vi "Parallel Processing (Optimized Performance).vi"() -> ()   [LabVIEW 2023]
doc: "The Parallel Processing (Optimized Performance) example shows how to process multiple images in parallel when using a ring acquisition. Images acquired from a camera are stored in a ring buffer and references to each image are pushed to a queue. Each worker loop removes a reference from the queue and processes the image.\n\nIn this example, image processing is simulated by a time delay that can be adjusted while the VI is running. When processing is complete, <B>IMAQdx Release Image</B> must be called in order to free space in the ring buffer."
uses:
  <vilib>/vision/driver/IMAQdx.llb/IMAQdx Acquisition Mode.ctl
  <vilib>/vision/Image Controls.llb/IMAQ Image.ctl
  <vilib>/vision/driver/IMAQdx.llb/IMAQdx Buffer Number Mode.ctl
  <vilib>/vision/driver/NI_Vision_Acquisition_Software.lvlib
  <resource>/objmgr/imaqdx.rc
panel:
  out "Lost Buffer Count":u32
  in  "Processing Delay (s)":dbl(slide)=0.1 scale=0.0..1.0
  out "Images Processed":u32
  out "Current Buffer Number":u32
  in  "Processing Delay (s)":dbl(slide)=0.2 scale=0.0..1.0
  out "Images Processed":u32
  out "Current Buffer Number":u32
  in  "Number of Images":i32=30
  out "Images in Queue":i32
  in  "Processing Delay (s)":dbl(slide)=0.4 scale=0.0..1.0
  out "Images Processed":u32
  out "Current Buffer Number":u32
  in  "Camera Name":refnum<k21> caption="IMAQdx Session"
  in  "Stop":bool
  # "Overview: Demonstrates how to process multiple extracted images in parallel when using a ring acquisition.\nRequirements: Vision Acquisition Software\nInstructions:\n1. Select the Camera Name\n2. Run the VI"
  # "Worker Loop 3"
  # "Worker Loop 2"
  # "Worker Loop 1"
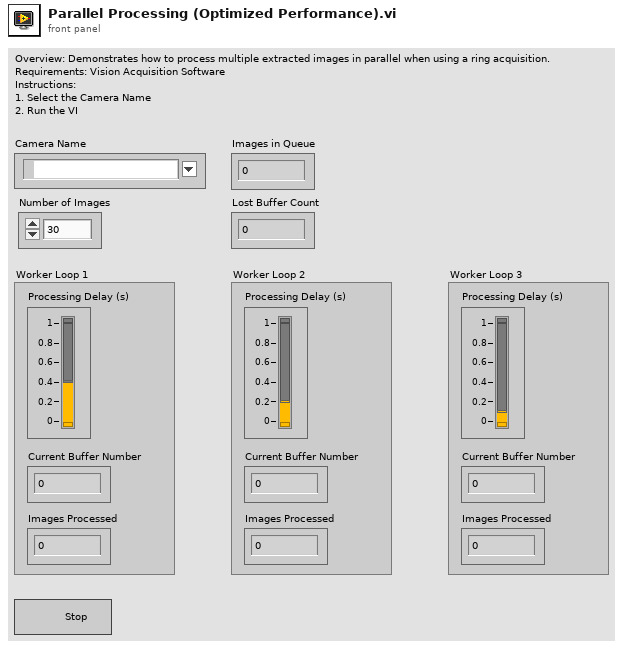
[diagram p1: front panel]
types:
  T1 = typedef "IMAQ Image.ctl" = refnum<image>
  T2 = typedef "NI_Vision_Acquisition_Software.lvlib/IMAQdx Acquisition Mode.ctl" = enum32{"One Shot", "Continuous"}
  T3 = typedef "IMAQdx.ctl" = refnum<k21>
  T4 = typedef "NI_Vision_Acquisition_Software.lvlib/IMAQdx Buffer Number Mode.ctl" = enum32{"Next", "Last", "Buffer Number", "Every", "Last New"}
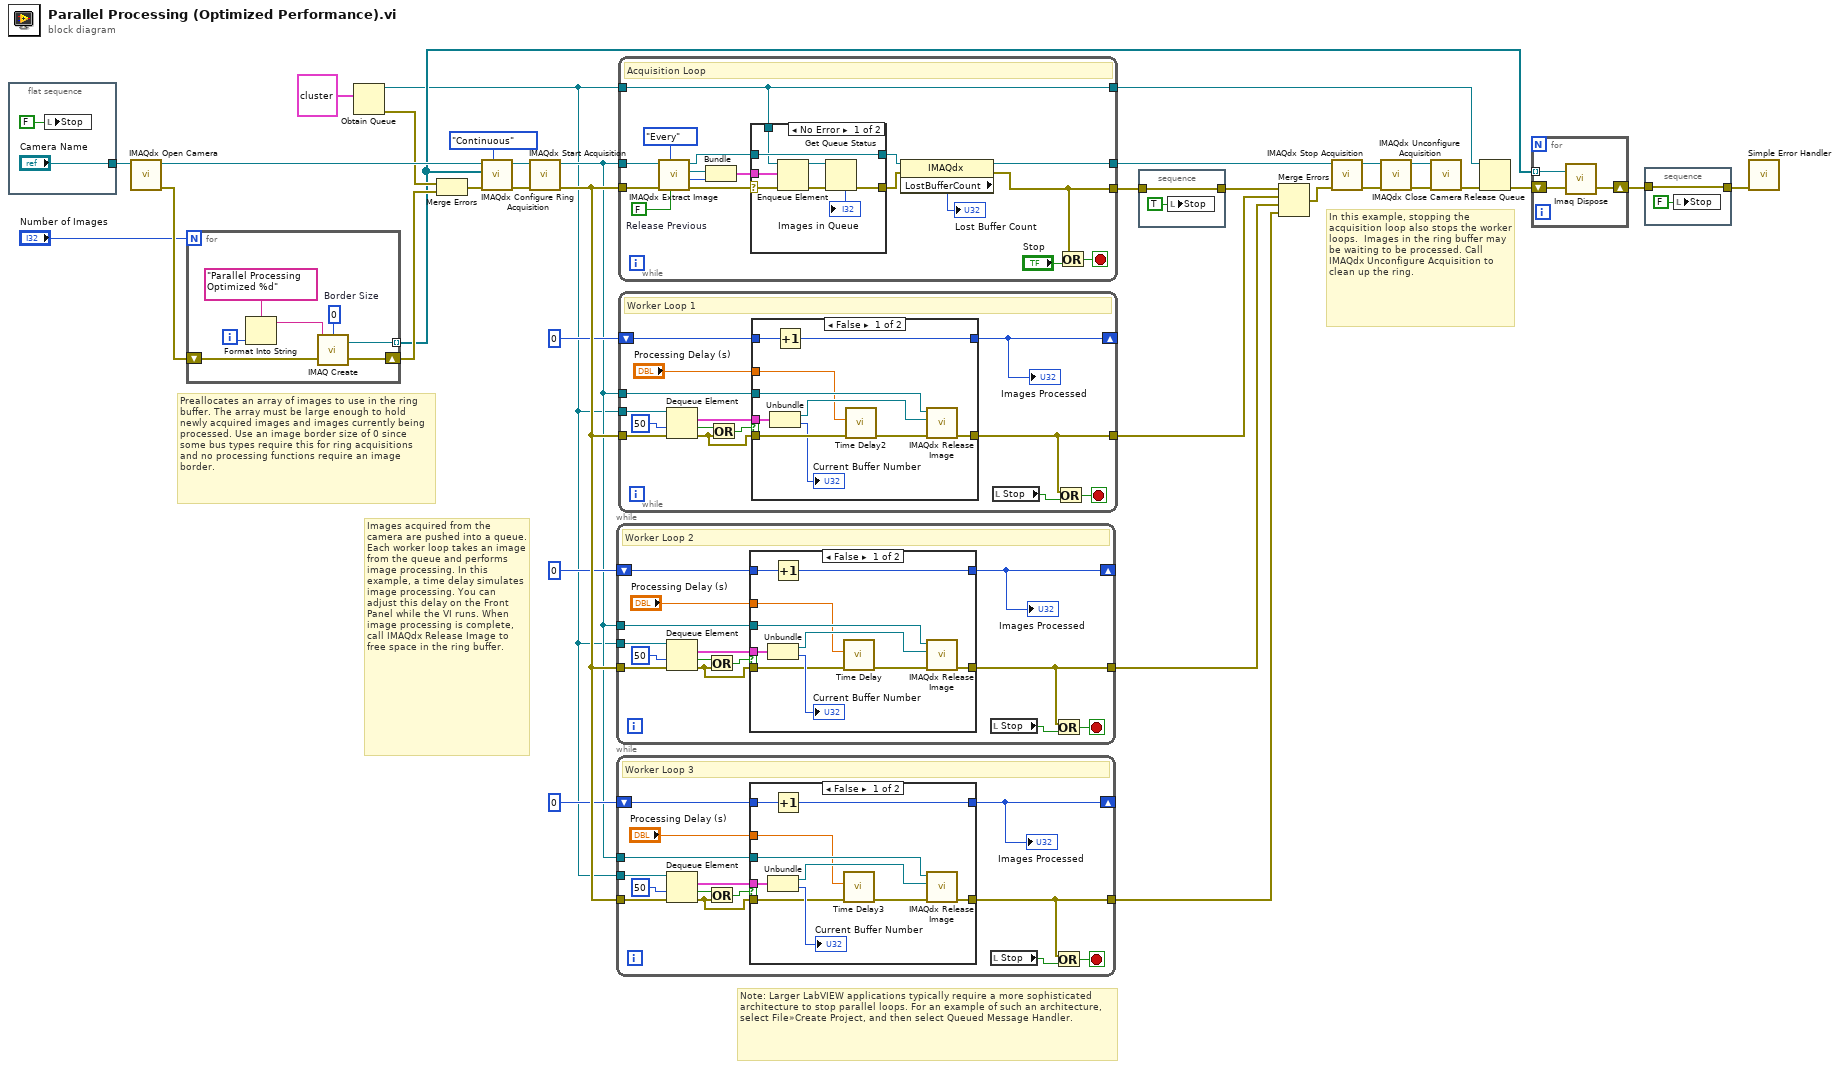
[diagram p0: block diagram]
diagram:
  # "In this example, stopping the acquisition loop also stops the worker loops.  Images in the ring buffer may be waiting to be processed. Call IMAQdx Unconfigure Acquisition to clean up the ring."
  # "Images acquired from the camera are pushed into a queue. Each worker loop takes an image from the queue and performs image processing. In this example, a time delay simulates image processing. You can adjust this delay on the Front Panel while the VI runs. When image processing is complete, call IMAQdx Release Image to free space in the ring buffer."
  # "Preallocates an array of images to use in the ring buffer. The array must be large enough to hold newly acquired images and images currently being processed. Use an image border size of 0 since some bus types require this for ring acquisitions and no processing functions require an image border."
  # "Note: Larger LabVIEW applications typically require a more sophisticated architecture to stop parallel loops. For an example of such an architecture, select File»Create Project, and then select Queued Message Handler."
  n1 = flat-sequence {
    tunnel: ["Camera Name"] -> w30
    frame #0 {
      n2 = local write "Stop"(FALSE ("Stop")) -> ()
    }
  }
  n3 = call <vilib>:"IMAQdx Open Camera.vi"("Session In"=w30) -> ("error out"=w23:errorcluster, "Session Out"=w22:T3)  [unwired: 2 in, 7 out]
  n4 = for {
    N: "Number of Images" -> [_]
    tunnel: [w42] -> w12 mode=indexing
    shift-right: [w41] -> w18
    shift-left: w23 -> [w43]
    i -> [w40]
    w37 = 0  # Border Size
    n5 = Format Into String(format string="Parallel Processing Optimized %d" ("Image Name"), w40) -> (resulting string=w39:string)  [unwired: 2 in, 1 out]
    n6 = call "IMAQ Create"("Border Size"=w37, "Image Name"=w39, "error in (no error)"=w43) -> ("New Image"=w42:T1, "error out"=w41:errorcluster)  [unwired: 1 in, 1 out]
  }
  n7 = Obtain Queue(element data type=cluster{"Image Out":T1, "Buffer Number Out":u32} {"Image Out"=refnum, "Buffer Number Out"=0}) -> (queue out=w5:refnum<queue>, error out=w17:errorcluster)  [unwired: 4 in, 1 out]
  n8 = Merge Errors(w17, w18) -> (w19:errorcluster)
  n9 = call <vilib>:"IMAQdx Configure Ring Acquisition.vi"("Mode"=IMAQdx_Acquisition_Mode."Continuous" ("Continuous?"), "error in"=w19, "Images"=w12, "Session In"=w22) -> ("error out"=w24:errorcluster, "Session Out"=w25:T3)  [unwired: 5 in, 1 out]
  n10 = call <vilib>:"IMAQdx Start Acquisition.vi"("error in"=w24, "Session In"=w25) -> ("error out"=w34:errorcluster, "Session Out"=w8:T3)  [unwired: 8 out]
  n11 = while {
    tunnel: [w50] -> w7
    tunnel: w5 -> [w54]
    tunnel: w8 -> [w53]
    shift-right: [w48] -> _
    shift-left: u32 0 -> [w52]
    tunnel: w34 -> [w47]
    stop <- w56 stop-if-true
    # "Worker Loop 2"
    n12 = Dequeue Element(queue=w54, timeout in ms (-1)=50 ("timeout in ms"), error in (no error)=w47) -> (element=w55:cluster{"Image Out":T1, "Buffer Number Out":u32}, timed out?=w44:bool, error out=w45:errorcluster)  [unwired: 1 out]
    n13 = Or(x=w44, y=w45) -> (x .or. y?=w46:bool)
    n14 = case shown="False" w46 {
      tunnel: w55 -> [w67 _]
      tunnel: [w66 w68] -> w50
      tunnel: "Processing Delay (s)" -> [w60 _]
      tunnel: w53 -> [w63 _]
      tunnel: w52 -> [w62 w69]
      tunnel: [w61 w69] -> w48
      tunnel: w45 -> [w58 w68]
      frame False {
        n15 = Unbundle(w67) -> ("Image Out"=w64:T1, "Buffer Number Out"=→"Current Buffer Number":u32)
        n16 = Increment(x=w62) -> (x+1=w61:u32)
        n17 = call "Time Delay"("error in (no error)"=w58, "Delay Time (s)"=w60) -> ("error out"=w65:errorcluster)  [unwired: 9 in]
        n18 = call <vilib>:"IMAQdx Release Image.vi"("error in"=w65, "Image"=w64, "Session In"=w63) -> ("error out"=w66:errorcluster)  [unwired: 7 in, 1 out]
      }
      frame True {
        # "Empty queue or error.\nNothing to process."
      }
    }
    "Images Processed" <- w48
    n19 = local read "Stop"() -> (w51:bool)
    n20 = Or(x=w50, y=w51) -> (x .or. y?=w56:bool)
  }
  n21 = while {
    tunnel: [w76] -> w6
    tunnel: w5 -> [w80]
    tunnel: w8 -> [w79]
    shift-right: [w74] -> _
    shift-left: u32 0 -> [w78]
    tunnel: w34 -> [w73]
    stop <- w82 stop-if-true
    # "Worker Loop 3"
    n22 = Dequeue Element(queue=w80, timeout in ms (-1)=50 ("timeout in ms"), error in (no error)=w73) -> (element=w81:cluster{"Image Out":T1, "Buffer Number Out":u32}, timed out?=w72:bool, error out=w70:errorcluster)  [unwired: 1 out]
    n23 = Or(x=w72, y=w70) -> (x .or. y?=w71:bool)
    n24 = case shown="False" w71 {
      tunnel: w81 -> [w93 _]
      tunnel: [w92 w94] -> w76
      tunnel: "Processing Delay (s)" -> [w86 _]
      tunnel: w79 -> [w89 _]
      tunnel: w78 -> [w88 w95]
      tunnel: [w87 w95] -> w74
      tunnel: w70 -> [w84 w94]
      frame False {
        n25 = Unbundle(w93) -> ("Image Out"=w90:T1, "Buffer Number Out"=→"Current Buffer Number":u32)
        n26 = Increment(x=w88) -> (x+1=w87:u32)
        n27 = call "Time Delay3"("error in (no error)"=w84, "Delay Time (s)"=w86) -> ("error out"=w91:errorcluster)  [unwired: 9 in]
        n28 = call <vilib>:"IMAQdx Release Image.vi"("error in"=w91, "Image"=w90, "Session In"=w89) -> ("error out"=w92:errorcluster)  [unwired: 7 in, 1 out]
      }
      frame True {
        # "Empty queue or error.\nNothing to process."
      }
    }
    "Images Processed" <- w74
    n29 = local read "Stop"() -> (w77:bool)
    n30 = Or(x=w76, y=w77) -> (x .or. y?=w82:bool)
  }
  n31 = while {
    tunnel: w34 -> [w112]
    tunnel: w8 -> [w108]
    tunnel: w5 -> [w97]
    tunnel: [w107] -> w11
    tunnel: [w105] -> w4
    tunnel: [w97] -> w13
    stop <- w104 stop-if-true
    w109 = FALSE  # Release Previous
    # "Acquisition Loop"
    n32 = call <vilib>:"IMAQdx Extract Image.vi"("Release Previous (true)"=w109, "Buffer Number Mode (Next)"=IMAQdx_Buffer_Number_Mode."Every" ("Buffer Number Mode"), "error in"=w112, "Session In"=w108) -> ("error out"=w103:errorcluster, "Buffer Number Out"=w102:u32, "Image Out"=w101:T1, "Session Out"=w100:T3)  [unwired: 4 in]
    n33 = Bundle("Image Out"=w101, "Buffer Number Out"=w102) -> (w98:cluster{"Image Out":T1, "Buffer Number Out":u32})  [unwired: 1 in]
    n34 = case shown="No Error" w103 {
      selector: w103 -> [w116 w121]
      tunnel: [w117 w122] -> w99
      tunnel: w100 -> [w117 w122]
      tunnel: w98 -> [w115 _]
      tunnel: w97 -> [w114 _]
      tunnel: [w113 w121] -> w96
      frame No Error {
        n35 = Enqueue Element(queue=w114, element=w115, error in (no error)=w116) -> (queue out=w119:refnum<queue>, error out=w120:errorcluster)  [unwired: 1 in, 1 out]
        n36 = Get Queue Status(queue=w119, error in (no error)=w120) -> (error out=w113:errorcluster, # elements in queue=→"Images in Queue":i32)  [unwired: 1 in, 6 out]
      }
      frame Error {
      }
    }
    n37 = property class="IMAQdx"(reference=w99, error in=w96) -> (reference out=w107:T3, error out=w105:errorcluster, "LostBufferCount"=→"Lost Buffer Count":u32)
    n38 = Or(x=w105, y="Stop") -> (x .or. y?=w104:bool)
  }
  n39 = while {
    tunnel: [w128] -> w14
    tunnel: w5 -> [w132]
    tunnel: w8 -> [w131]
    shift-right: [w127] -> _
    shift-left: u32 0 -> [w130]
    tunnel: w34 -> [w126]
    stop <- w135 stop-if-true
    # "Worker Loop 1"
    n40 = Dequeue Element(queue=w132, timeout in ms (-1)=50 ("timeout in ms"), error in (no error)=w126) -> (element=w134:cluster{"Image Out":T1, "Buffer Number Out":u32}, timed out?=w124:bool, error out=w123:errorcluster)  [unwired: 1 out]
    n41 = Or(x=w124, y=w123) -> (x .or. y?=w125:bool)
    n42 = case shown="False" w125 {
      tunnel: w123 -> [w143 w148]
      tunnel: w134 -> [w146 _]
      tunnel: [w145 w148] -> w128
      tunnel: "Processing Delay (s)" -> [w137 _]
      tunnel: w131 -> [w141 _]
      tunnel: w130 -> [w139 w147]
      tunnel: [w138 w147] -> w127
      frame False {
        n43 = Unbundle(w146) -> ("Image Out"=w142:T1, "Buffer Number Out"=→"Current Buffer Number":u32)
        n44 = Increment(x=w139) -> (x+1=w138:u32)
        n45 = call "Time Delay2"("error in (no error)"=w143, "Delay Time (s)"=w137) -> ("error out"=w144:errorcluster)  [unwired: 9 in]
        n46 = call <vilib>:"IMAQdx Release Image.vi"("error in"=w144, "Image"=w142, "Session In"=w141) -> ("error out"=w145:errorcluster)  [unwired: 7 in, 1 out]
      }
      frame True {
        # "Empty queue or error.\nNothing to process."
      }
    }
    "Images Processed" <- w127
    n47 = local read "Stop"() -> (w129:bool)
    n48 = Or(x=w128, y=w129) -> (x .or. y?=w135:bool)
  }
  n49 = stacked-sequence {
    tunnel: [w149] -> w3
    tunnel: w4 -> [w149]
    frame #0 {
      n50 = local write "Stop"(TRUE ("Stop")) -> ()
    }
  }
  n51 = Merge Errors(w3, w14, w7, w6) -> (w16:errorcluster)
  n52 = call <vilib>:"IMAQdx Stop Acquisition.vi"("error in"=w16, "Session In"=w11) -> ("error out"=w26:errorcluster, "Session Out"=w27:T3)  [unwired: 8 out]
  n53 = call <vilib>:"IMAQdx Unconfigure Acquisition.vi"("error in"=w26, "Session In"=w27) -> ("error out"=w29:errorcluster, "Session Out"=w28:T3)  [unwired: 8 out]
  n54 = call <vilib>:"IMAQdx Close Camera.vi"("error in"=w29, "Session In"=w28) -> ("error out"=w10:errorcluster)  [unwired: 9 out]
  n55 = Release Queue(queue=w13, error in (no error)=w10) -> (error out=w9:errorcluster)  [unwired: 1 in, 2 out]
  n56 = for {
    shift-right: [w152] -> w2
    shift-left: w9 -> [w153]
    tunnel: w12 -> [w151] mode=indexing
    n57 = call "Imaq Dispose"("Image"=w151, "error in (no error)"=w153) -> ("error out"=w152:errorcluster)  [unwired: 4 in]
  }
  n58 = stacked-sequence {
    tunnel: [w154] -> w1
    tunnel: w2 -> [w154]
    frame #0 {
      n59 = local write "Stop"(FALSE ("Stop")) -> ()
    }
  }
  n60 = call <vilib>:"Simple Error Handler.vi"("error in (no error)"=w1) -> ()  [unwired: 4 in, 5 out]
